vi "Event Handle Loop_Delete Button.vi"(8 "error in (no error)":errorcluster, 11 "QMenu Class in":refnum<class "QMenu Class.lvclass">) -> (0 "error out":errorcluster, 3 "QMenu Class out":refnum<class "QMenu Class.lvclass">)   [LabVIEW 2020, in "QTab.lvlib" / "QMenu Class.lvclass"]
uses:
  QMenu Class.lvclass
  QMenu Class.lvclass/QMenu Class.ctl
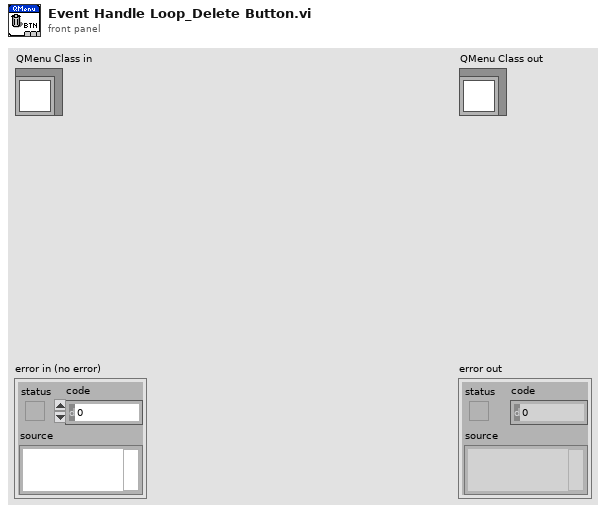
[diagram p1: front panel]
types:
  T1 = typedef "QTab.lvlib/QMenu Class.lvclass/Button Attribute.ctl" = cluster{"Label":string, "Button Text":string, "Closable":bool, "Draggable":bool}
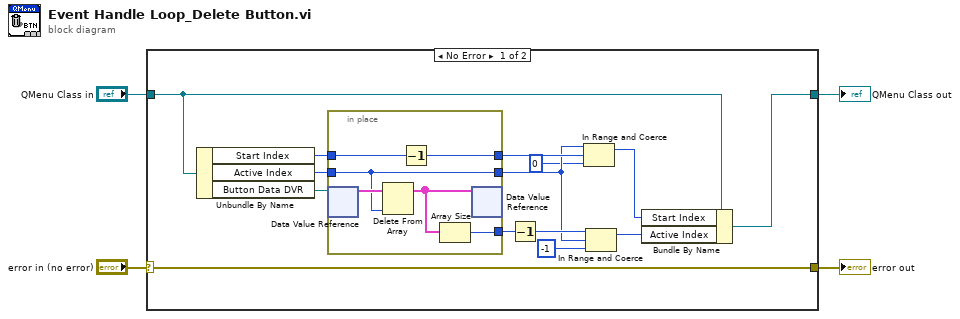
[diagram p0: block diagram]
diagram:
  n1 = case shown="No Error" "error in (no error)" {
    selector: "error in (no error)" -> [w6 w25]
    tunnel: "QMenu Class in" -> [w7 w26]
    tunnel: [w6 w25] -> w1
    tunnel: [w5 w26] -> w2
    frame No Error {
      n2 = Unbundle By Name(w7) -> ("Start Index"=w13:i32, "Active Index"=w17:i32, "Button Data DVR"=w18:refnum<data-value>)
      n3 = in-place {
        in-place-border: w17 -> [w23]
        in-place-border: [w23] -> w10
        in-place-border: [w21] -> w15
        in-place-border: w13 -> [w20]
        in-place-border: [w19] -> w12
        n4 = in-place-dvr #1(w18) -> (w24:T1[])  [unwired: 1 out]
        n5 = Delete From Array(array=w24, index=w23) -> (array with subset deleted=w22:T1[])  [unwired: 1 in, 1 out]
        n6 = Decrement(x=w20) -> (x-1=w19:i32)
        n7 = Array Size(array=w22) -> (size(s)=w21:i32)
        n8 = in-place-dvr #1(w22) -> ()  [unwired: 2 out]
      }
      n9 = Decrement(x=w15) -> (x-1=w14:i32)
      n10 = In Range and Coerce(upper limit=w10, x=w12, lower limit=0) -> (coerced(x)=w9:i32)  [unwired: 1 out]
      n11 = In Range and Coerce(upper limit=w14, x=w10, lower limit=-1) -> (coerced(x)=w16:i32)  [unwired: 1 out]
      n12 = Bundle By Name(cluster=w7, "Start Index"=w9, "Active Index"=w16) -> (w5:refnum<class "QMenu Class.lvclass">)
    }
    frame Error {
    }
  }
  "error out" <- w1
  "QMenu Class out" <- w2
